vi "Read data.vi"(8 "error in (no error)":errorcluster, 10 "Buffer mode":T1, 11 "Scope5785_six_channel":refnum<class "Scope5782_six_channel.lvclass">) -> (0 "error out":errorcluster, 1 "Any read?":bool, 2 "Data":dbl[][](array[numeric]), 3 "Scope5785_six_channel out":refnum<class "Scope5782_six_channel.lvclass">, 4 "FFT buffer":dbl[][](array[numeric]))   [LabVIEW 2018, in "Scope5782_six_channel.lvclass"]
uses:
  Scope5782_six_channel.lvclass
  C:/PXIe/InProgress/source/Host/Scope/ScopeBase/ScopeBase.lvclass
  controls/Data_display_mode.ctl
  ScopeBase/ScopeBase.lvclass/ScopeBase.ctl
  ScopeBase/ScopeBase.lvclass
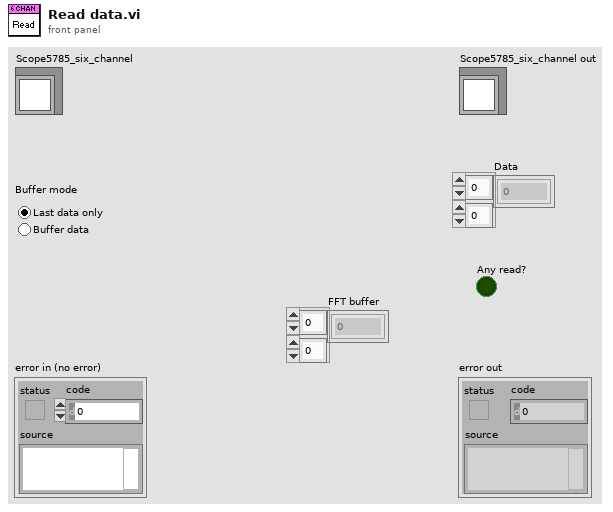
[diagram p1: front panel]
types:
  T1 = typedef "Data_display_mode.ctl" = enum32{"Last data only", "Buffer data"}
  T2 = typedef "ScopeMode.ctl" = enum16{"Stopped", "Single", "Running", "Continuous"}
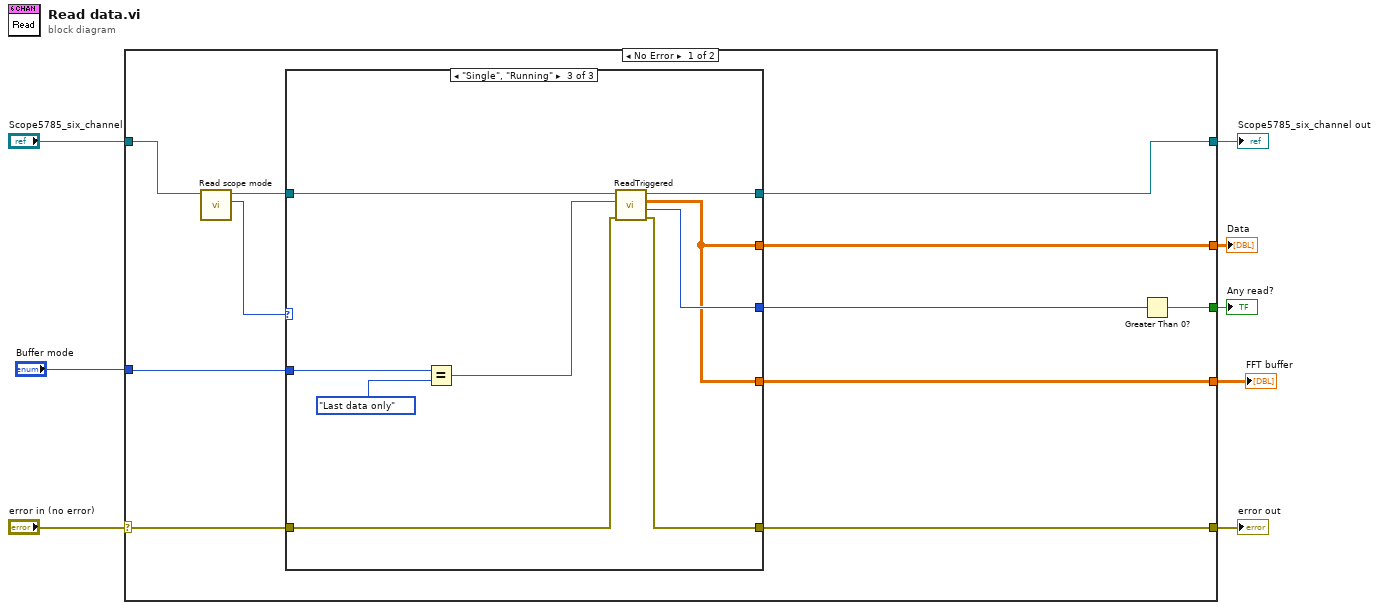
[diagram p0: block diagram]
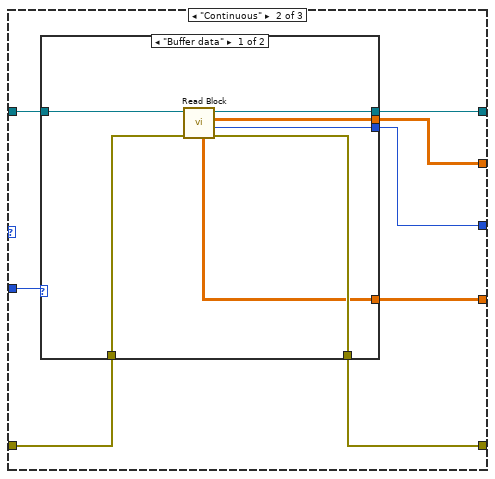
[diagram p3: hidden frame]
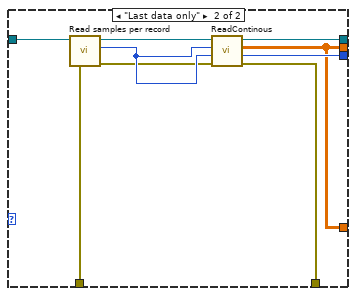
[diagram p4: hidden frame]
diagram:
  n1 = case shown="No Error" "error in (no error)" {
    selector: "error in (no error)" -> [w10 w55]
    tunnel: [w11 w55] -> w7
    tunnel: [w16 w54] -> w5
    tunnel: "Scope5785_six_channel" -> [w19 w54]
    tunnel: "Buffer mode" -> [w12 _]
    tunnel: [w15 _] -> w2
    tunnel: [w13 _] -> w3
    tunnel: [w9 _] -> w1
    frame No Error {
      n2 = call "Read scope mode.vi"("ScopeBase in"=w19) -> ("scope mode"=w17:T2, "ScopeBase out"=w18:refnum<class "Scope5782_six_channel.lvclass">)  [unwired: 8 in, 1 out]
      n3 = case shown="\"Single\", \"Running\"" w17 {
        tunnel: w18 -> [w21 w26 w53]
        tunnel: [w21 w29 w52] -> w16
        tunnel: [_ w28 w45] -> w15
        tunnel: [_ w27 w51] -> w14
        tunnel: w12 -> [_ w23 w49]
        tunnel: [w20 w24 w47] -> w11
        tunnel: w10 -> [w20 w25 w46]
        tunnel: [_ w22 w45] -> w9
        frame "Stopped", Default {
        }
        frame "Continuous" {
          n4 = case shown="\"Buffer data\"" w23 {
            tunnel: [w35 w44] -> w29
            tunnel: [w34 w37] -> w28
            tunnel: [w33 w43] -> w27
            tunnel: w26 -> [w36 w41]
            tunnel: w25 -> [w32 w39]
            tunnel: [w31 w38] -> w24
            tunnel: [w30 w37] -> w22
            frame "Buffer data" {
              n5 = call-dynamic "Read Block.vi"("error in (no error)"=w32, "Scope5761"=w36) -> ("error out"=w31:errorcluster, "#elements"=w33:i32, "Data"=w34:dbl[][], "Scope5761"=w35:refnum<class "Scope5782_six_channel.lvclass">, "FFT buffer"=w30:dbl[][])  [unwired: 5 in]
            }
            frame "Last data only" {
              n6 = call "Read samples per record.vi"("ScopeBase in"=w41) -> ("samples per record"=w42:i32, "ScopeBase out"=w40:refnum<class "Scope5782_six_channel.lvclass">)  [unwired: 8 in, 1 out]
              n7 = call-dynamic "ReadContinous.vi"("error in (no error)"=w39, "Max samples to keep"=w42, "Min samples to read"=w42, "Scope5785_six_channel"=w40) -> ("error out"=w38:errorcluster, "#elements"=w43:i32, "Data"=w37:dbl[][], "Scope5785_six_channel Out"=w44:refnum<class "Scope5782_six_channel.lvclass">)  [unwired: 4 in]
            }
          }
        }
        frame "Single", "Running" {
          n8 = Equal?(x=w49, y=Data_display_mode."Last data only") -> (x = y?=w48:bool)
          n9 = call-dynamic "ReadTriggered.vi"("error in (no error)"=w46, "Keep last record only"=w48, "Scope5785_six_channel"=w53) -> ("error out"=w47:errorcluster, "#elements"=w51:i32, "Data"=w45:dbl[][], "Scope5785_six_channel Out"=w52:refnum<class "Scope5782_six_channel.lvclass">)  [unwired: 5 in]
        }
      }
      n10 = Greater Than 0?(x=w14) -> (x > 0?=w13:bool)
    }
    frame Error {
    }
  }
  "error out" <- w7
  "Scope5785_six_channel out" <- w5
  "Any read?" <- w3
  "Data" <- w2
  "FFT buffer" <- w1
